vi "manual_test_comparison.vi"(5 "change_in_event":refnum<user-event>, 7 "waitgroup":T1, 8 "error in (no error)":errorcluster, 11 "data":variant) -> (0 "error out":errorcluster)   [LabVIEW 2015, in "example_01.lvlib"]
uses:
  example_01.lvlib
  <userlib>/antonio-alexander/lv-waitgroup/public/_controls/api_waitgroup.ctl
  lv-recipe-machine/public/_controls/change.ctl
  _controls/step_data.ctl
  _controls/manual_actions.ctl
  lv-recipe-machine/lv-recipe-machine.lvlib
  <userlib>/antonio-alexander/lv-waitgroup/lv-waitgroup.lvlib
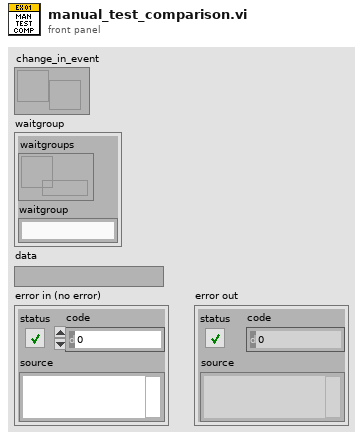
[diagram p1: front panel]
types:
  T1 = typedef "lv-waitgroup.lvlib/api_waitgroup.ctl" = cluster{"waitgroups":refnum<data-value>, "waitgroup":string}
  T2 = typedef "example_01.lvlib/manual_actions.ctl" = enum16{"<manual_action>", "manual_test_random", "manual_test_comparison", "manual_test_wait", "<null>"}
  T3 = typedef "example_01.lvlib/step_data.ctl" = cluster{"data":variant, "step":string}
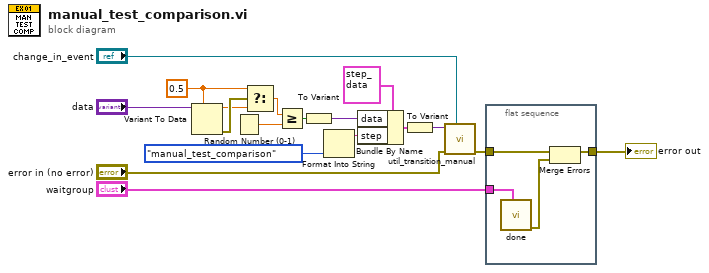
[diagram p0: block diagram]
diagram:
  w10 = 0.5
  n1 = Variant To Data(type=w10, Variant="data") -> (data=w9:dbl, error out=w11:errorcluster)  [unwired: 1 in]
  n2 = Random Number (0-1)() -> (number: 0 to 1=w12:dbl)
  n3 = Select(t=w10, s=w11, f=w9) -> (s? t:f=w8:dbl)
  n4 = Greater Or Equal?(x=w8, y=w12) -> (x >= y?=w7:bool)
  n5 = To Variant(anything=w7) -> (Variant=w14:variant)
  n6 = Format Into String(manual_actions."manual_test_comparison" ("manual_action")) -> (resulting string=w15:string)  [unwired: 3 in, 1 out]
  n7 = Bundle By Name(cluster=T3 {"data"=variant, "step"=""}, "data"=w14, "step"=w15) -> (w6:T3)
  n8 = To Variant(anything=w6) -> (Variant=w5:variant)
  n9 = call "util_transition_manual.vi"("change_in_event"="change_in_event", "error in (no error)"="error in (no error)", "data"=w5) -> ("error out"=w3:errorcluster)  [unwired: 8 in]
  n10 = flat-sequence {
    tunnel: "waitgroup" -> [w22]
    tunnel: w3 -> [w21]
    tunnel: [w20] -> w2
    frame #0 {
      n11 = call <userlib>:"done.vi"("waitgroup"=w22) -> ("error out"=w19:errorcluster)  [unwired: 10 in]
      n12 = Merge Errors(w21, w19) -> (w20:errorcluster)
    }
  }
  "error out" <- w2
